vi "ExceptionStacker.vi"(2 "ExceptionString":string, 7 "Newmark-Exceptions IN":T1={"Command Error"=TRUE, "Slip/Stall"=TRUE, "Overtravel"=TRUE, "Done"=TRUE, "nError"=0, "nSlip"=0, "nOT"=0, "nDone"=0}) -> (8 "Newmark-Exceptions OUT":T1={"Command Error"=TRUE, "Slip/Stall"=TRUE, "Overtravel"=TRUE, "Done"=TRUE, "nError"=0, "nSlip"=0, "nOT"=0, "nDone"=0})   [LabVIEW 2019]
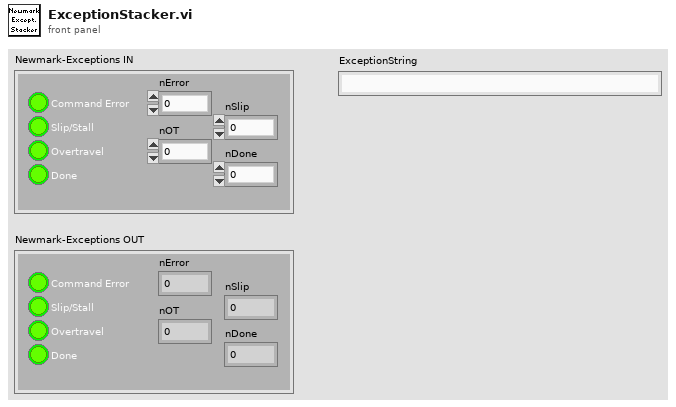
[diagram p1: front panel]
types:
  T1 = cluster{"Command Error":bool, "Slip/Stall":bool, "Overtravel":bool, "Done":bool, "nError":u32, "nSlip":u32, "nOT":u32, "nDone":u32}
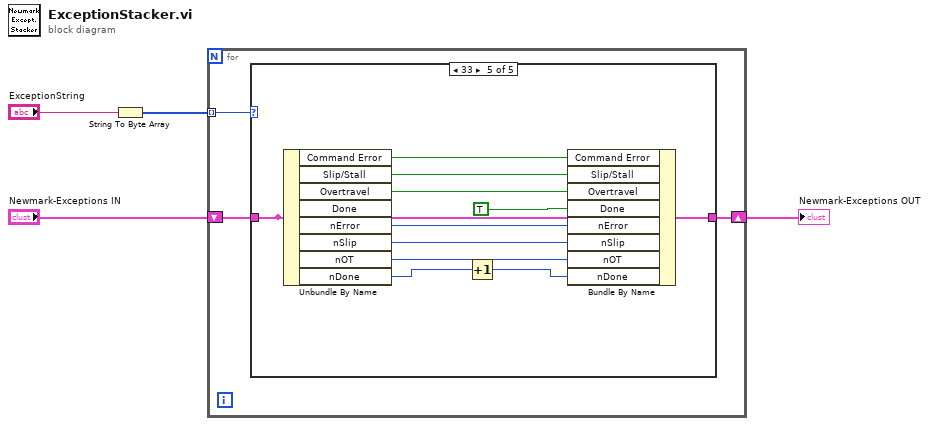
[diagram p0: block diagram]
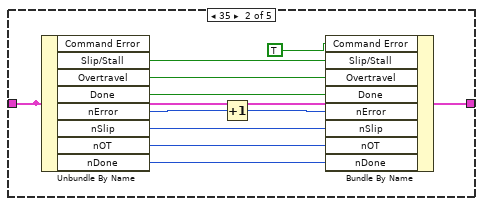
[diagram p3: hidden frame]
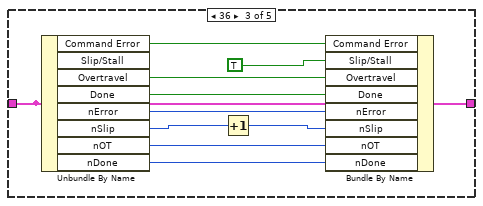
[diagram p4: hidden frame]
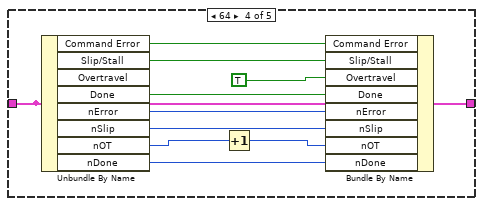
[diagram p5: hidden frame]
diagram:
  n1 = String To Byte Array(string="ExceptionString") -> (unsigned byte array=w3:u8[])
  n2 = for {
    tunnel: w3 -> [w7] mode=indexing
    shift-right: [w5] -> w1
    shift-left: "Newmark-Exceptions IN" -> [w6]
    n3 = case shown="33" w7 {
      tunnel: w6 -> [w8 w18 w29 w40 w51]
      tunnel: [w8 w19 w30 w41 w52] -> w5
      frame Default {
      }
      frame 35 {
        n4 = Unbundle By Name(w18) -> ("Slip/Stall"=w16:bool, "Overtravel"=w15:bool, "Done"=w14:bool, "nError"=w13:u32, "nSlip"=w11:u32, "nOT"=w10:u32, "nDone"=w9:u32)  [unwired: 1 out]
        n5 = Increment(x=w13) -> (x+1=w12:u32)
        n6 = Bundle By Name(cluster=w18, "Command Error"=TRUE, "Slip/Stall"=w16, "Overtravel"=w15, "Done"=w14, "nError"=w12, "nSlip"=w11, "nOT"=w10, "nDone"=w9) -> (w19:T1)
      }
      frame 36 {
        n7 = Unbundle By Name(w29) -> ("Command Error"=w24:bool, "Overtravel"=w28:bool, "Done"=w27:bool, "nError"=w22:u32, "nSlip"=w21:u32, "nOT"=w26:u32, "nDone"=w25:u32)  [unwired: 1 out]
        n8 = Increment(x=w21) -> (x+1=w20:u32)
        n9 = Bundle By Name(cluster=w29, "Command Error"=w24, "Slip/Stall"=TRUE, "Overtravel"=w28, "Done"=w27, "nError"=w22, "nSlip"=w20, "nOT"=w26, "nDone"=w25) -> (w30:T1)
      }
      frame 64 {
        n10 = Unbundle By Name(w40) -> ("Command Error"=w37:bool, "Slip/Stall"=w34:bool, "Done"=w39:bool, "nError"=w36:u32, "nSlip"=w33:u32, "nOT"=w32:u32, "nDone"=w38:u32)  [unwired: 1 out]
        n11 = Increment(x=w32) -> (x+1=w31:u32)
        n12 = Bundle By Name(cluster=w40, "Command Error"=w37, "Slip/Stall"=w34, "Overtravel"=TRUE, "Done"=w39, "nError"=w36, "nSlip"=w33, "nOT"=w31, "nDone"=w38) -> (w41:T1)
      }
      frame 33 {
        n13 = Unbundle By Name(w51) -> ("Command Error"=w49:bool, "Slip/Stall"=w47:bool, "Overtravel"=w44:bool, "nError"=w48:u32, "nSlip"=w46:u32, "nOT"=w43:u32, "nDone"=w50:u32)  [unwired: 1 out]
        n14 = Increment(x=w50) -> (x+1=w42:u32)
        n15 = Bundle By Name(cluster=w51, "Command Error"=w49, "Slip/Stall"=w47, "Overtravel"=w44, "Done"=TRUE, "nError"=w48, "nSlip"=w46, "nOT"=w43, "nDone"=w42) -> (w52:T1)
      }
    }
  }
  "Newmark-Exceptions OUT" <- w1
